vi "Read position.vi"(8 "error in (no error)":errorcluster, 11 "Bomb in":refnum<class "Bomb.lvclass">) -> (0 "error out":errorcluster, 2 "position":cluster{"x":dbl, "y":dbl}, 3 "Bomb out":refnum<class "Bomb.lvclass">)   [LabVIEW 2021]
uses:
  Bomb.lvclass
  C:/Users/poche/Programs/LabVIEW/Snake Game/GameEl_class/GameEl.lvclass
  C:/Users/poche/Programs/LabVIEW/Snake Game/Bomb/Bomb.lvclass
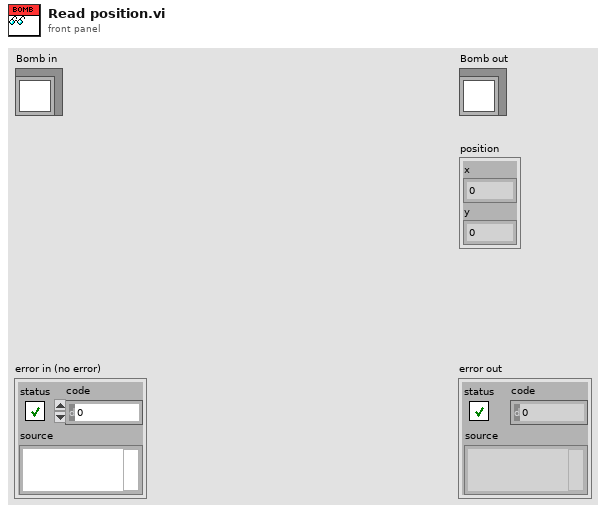
[diagram p1: front panel]
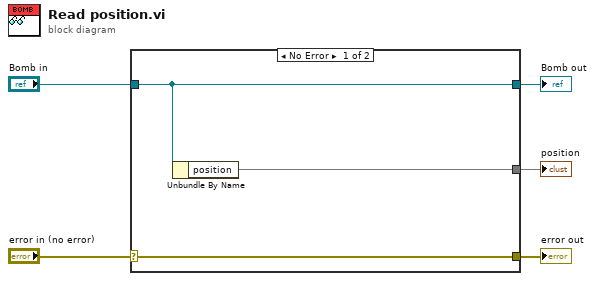
[diagram p0: block diagram]
diagram:
  n1 = case shown="No Error" "error in (no error)" {
    selector: "error in (no error)" -> [w8 w9]
    tunnel: [w8 w9] -> w4
    tunnel: [w7 w10] -> w2
    tunnel: "Bomb in" -> [w7 w10]
    tunnel: [w6 _] -> w1
    frame No Error {
      n2 = Unbundle By Name(w7) -> ("position"=w6)
    }
    frame Error {
    }
  }
  "error out" <- w4
  "Bomb out" <- w2
  "position" <- w1
